vi "Global_Sample per Frame.vi"() -> ()   [LabVIEW 2015]
panel:
  in  "Imaging data averaged":u32
  in  "Imaging data unpacked for Kalman":u32
  in  "Imaging data DRAM address":u32
  in  "Max DRAM address":u32
  in  "Waveform output loop count":i32
  in  "Num of elements":u32=512000
  in  "Num of data":u32
  in  "Display imaging data address":u32
  in  "Kalman Imaging data address":u32
  in  "Galvo signal readed":u32
  in  "Frames done":i32
  in  "Number of frames":i32
  out "Samples acquired":u32
  in  "SubVi Indicator":i32
  in  "image data address indicator":u32
  in  "Address counter":u32
  in  "Data":u32
  out "Averaged image displayed?_Global":bool
  out "Frame acquisition finish?_Global":bool
  out "Frame address_Global":u32
  in  "Samples per frame_Global":u32
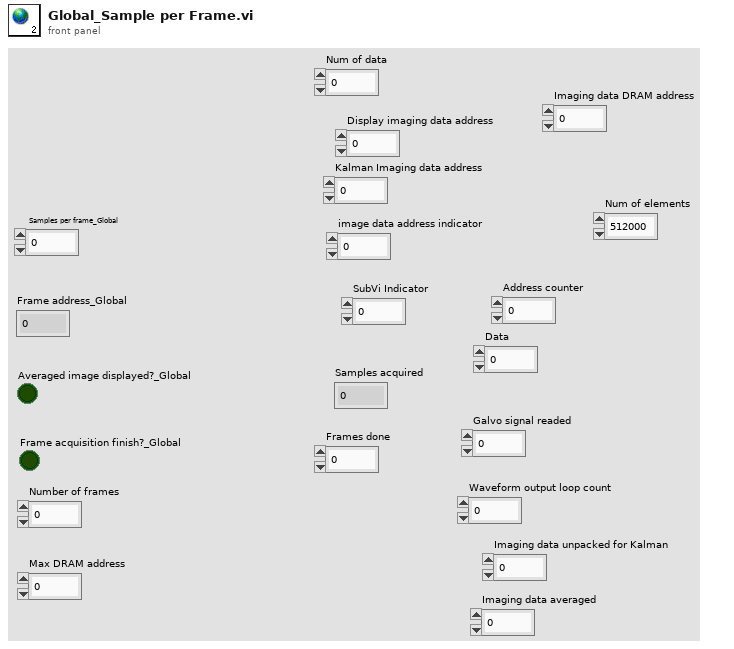
[diagram p1: front panel]
diagram:
